vi "TolCheck.vi"(7 "Tol. Sup.:":sgl min=0, 8 "error in (no error)":errorcluster, 9 "Tol. Inf.:":sgl max=0, 10 "Pre. TI:":sgl max=0, 11 "Pre. TS:":sgl min=0) -> (0 "error out":errorcluster, 1 "Tol. Inf.:":sgl max=0, 2 "Pre. TI:":sgl max=0, 3 "Pre. TS:":sgl min=0, 5 "Tol. Sup.:":sgl min=0)   [LabVIEW 2014, in "ConfigProg.lvlib"]
doc: "Chequea que las Pre-tolerancias no superen a las Tolerancias."
uses:
  ConfigProg.lvlib
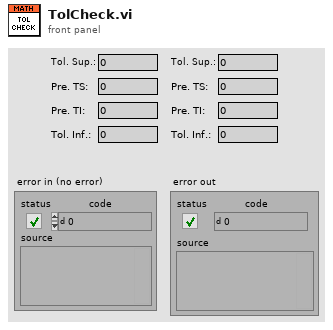
[diagram p1: front panel]
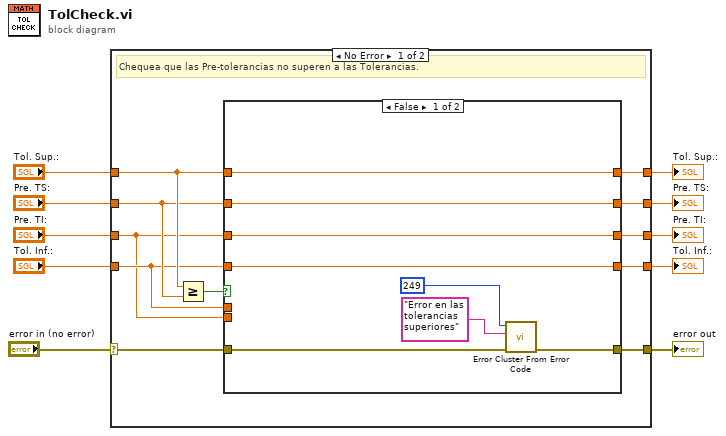
[diagram p0: block diagram]
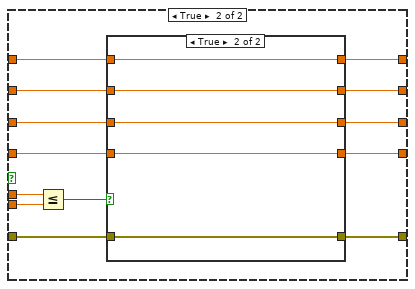
[diagram p2: hidden frame]
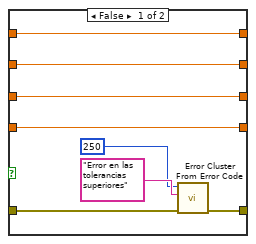
[diagram p3: hidden frame]
diagram:
  n1 = case shown="No Error" "error in (no error)" {
    selector: "error in (no error)" -> [w11 w60]
    tunnel: "Tol. Sup.:" -> [w20 w59]
    tunnel: "Pre. TS:" -> [w19 w58]
    tunnel: "Tol. Inf.:" -> [w18 w56]
    tunnel: "Pre. TI:" -> [w17 w57]
    tunnel: [w16 w59] -> w6
    tunnel: [w15 w58] -> w5
    tunnel: [w14 w57] -> w4
    tunnel: [w13 w56] -> w3
    tunnel: [w12 w60] -> w2
    frame No Error {
      # "Chequea que las Pre-tolerancias no superen a las Tolerancias."
      n2 = Greater Or Equal?(x=w20, y=w19) -> (x >= y?=w21:bool)
      n3 = case shown="False" w21 {
        tunnel: [w29 w41] -> w16
        tunnel: [w28 w40] -> w15
        tunnel: [w27 w39] -> w14
        tunnel: [w26 w38] -> w13
        tunnel: w18 -> [_ w37]
        tunnel: w17 -> [_ w36]
        tunnel: w20 -> [w29 w35]
        tunnel: w19 -> [w28 w34]
        tunnel: w17 -> [w27 w33]
        tunnel: w18 -> [w26 w32]
        tunnel: [w24 w31] -> w12
        tunnel: w11 -> [w25 w30]
        frame False {
          n4 = call <vilib>:"Error Cluster From Error Code.vi"("error in (no error)"=w25, "error message (\"\")"="Error en las tolerancias superiores" ("error message (\"\")"), "error code (0)"=249) -> ("error out"=w24:errorcluster)  [unwired: 6 in]
        }
        frame True {
          n5 = Less Or Equal?(x=w37, y=w36) -> (x <= y?=w42:bool)
          n6 = case shown="True" w42 {
            tunnel: [w48 w55] -> w41
            tunnel: [w47 w54] -> w40
            tunnel: [w46 w53] -> w39
            tunnel: [w45 w52] -> w38
            tunnel: w35 -> [w48 w55]
            tunnel: w34 -> [w47 w54]
            tunnel: w33 -> [w46 w53]
            tunnel: w32 -> [w45 w52]
            tunnel: [w49 w51] -> w31
            tunnel: w30 -> [w50 w51]
            frame False {
              n7 = call <vilib>:"Error Cluster From Error Code.vi"("error in (no error)"=w50, "error message (\"\")"="Error en las tolerancias superiores" ("error message (\"\")"), "error code (0)"=250) -> ("error out"=w49:errorcluster)  [unwired: 6 in]
            }
            frame True {
            }
          }
        }
      }
    }
    frame Error {
    }
  }
  "Tol. Sup.:" <- w6
  "Pre. TS:" <- w5
  "Pre. TI:" <- w4
  "Tol. Inf.:" <- w3
  "error out" <- w2
